vi "Acceleration Sensor-Dual.vi"() -> ()   [LabVIEW 2009]
uses:
  <vilib>/NXT/Block Support/NXT_InputPort.ctl
  <vilib>/NXT/Subs/LVHSConnector.ctl
  mindsensors.com LVEE Toolkit/Dual/Acceleration Sensor-DM.vi
panel:
  out "Status (boolean)":bool
  in  "stop":bool
  out "Z":i16(knob)=231 scale=-2000.0..2000.0
  out "Y":i16(knob) scale=-2000.0..2000.0
  out "X":i16(knob)=234 scale=-2000.0..2000.0
  out "X":i16(slide)=126 scale=-35.0..35.0
  out "Z":i16(slide)=129 caption="Y" scale=-35.0..35.0
  out "Y":i16(slide)=128 scale=-35.0..35.0
  out "Z":i16(slide)=125 caption="X" scale=-35.0..35.0
  out "Y 3":i16(slide)=128 caption="Y" scale=-35.0..35.0
  out "X":i16(slide)=126 scale=-35.0..35.0
  out "Z":dbl
  out "Y":dbl
  out "X":dbl
  out "Z":dbl=128.0
  out "Y  5":dbl=128.0
  out "X":dbl=128.0
  out "NXT dup":T1={"error"={"status"=FALSE, "code"=0, "source"=""}, "address"="", "NXT #"=-1, "Show Error"=TRUE} caption="NXT"
  in  "NXT":T1={"error"={"status"=FALSE, "code"=0, "source"=""}, "address"="", "NXT #"=-1, "Show Error"=TRUE}
  in  "Input Port":T2 items=["Port 1", "Port 2", "Port 3", "Port 4"]
  # "Tilt"
  # "Acceleration"
  # "mindsensors.com\nCopyright (c) 2009 by mindsensors.com\nEmail: info (<at>) mindsensors (<dot>) com\n\nThis program is free software. You can redistribute it and/or modify\nit under the terms of the GNU General Public License as published by\nthe Free Software Foundation; version 3 of the License.\nRead the license at: http://www.gnu.org/licenses/gpl.txt"
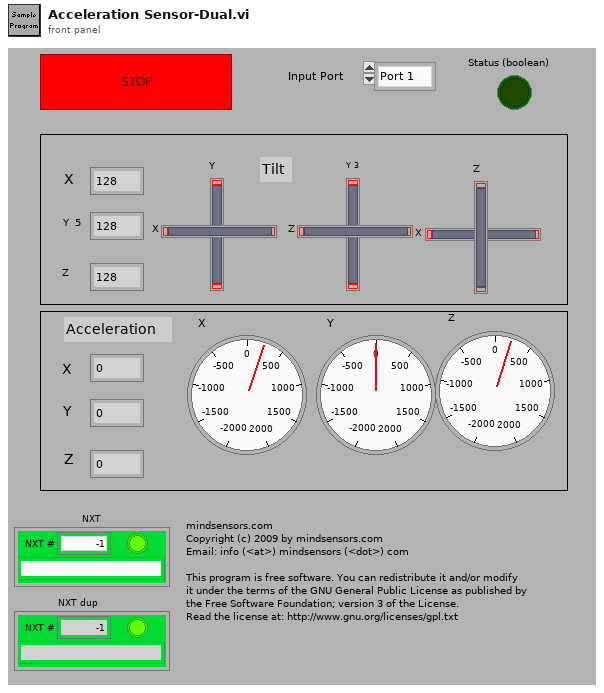
[diagram p1: front panel]
types:
  T1 = typedef "LVHSConnector.ctl" = cluster{"error":errorcluster, "address":string, "NXT #":i32, "Show Error":bool}
  T2 = typedef "NXT_InputPort.ctl" = u8
  T3 = cluster{"X Tilt":i16, "Y Tilt":i16, "Z Tilt":i16, "X Accel":i16, "Y Accel":i16, "Z Accel":i16, "Status (boolean)":bool}
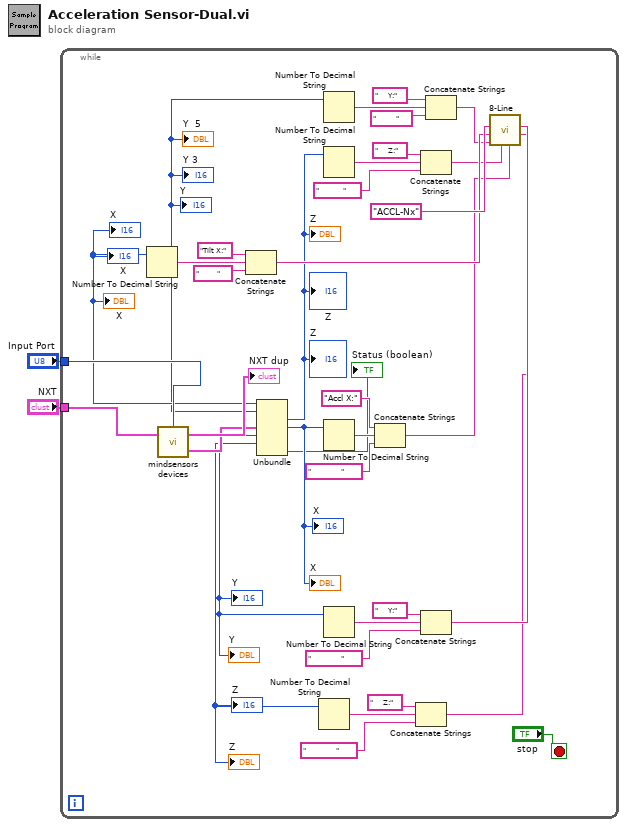
[diagram p0: block diagram]
diagram:
  n1 = while {
    tunnel: "Input Port" -> [w14]
    tunnel: "NXT" -> [w13]
    stop <- "stop" stop-if-true
    n2 = call-poly "mindsensors devices.vi"("NXT"=w13, "Input Port"=w14) -> ("Output of Acceleration Sensor"=w11:T3, "NXT dup"=→"NXT dup":T1)  [unwired: 1 in]
    n3 = Unbundle(w11) -> ("X Tilt"=w10:i16, "Y Tilt"=w9:i16, "Z Tilt"=w8:i16, "X Accel"=w7:i16, "Y Accel"=w6:i16, "Z Accel"=w5:i16, "Status (boolean)"=→"Status (boolean)":bool)
    "X" <- w10
    "Y  5" <- w9
    "Z" <- w8
    "X" <- w7
    "Y" <- w6
    "Z" <- w5
    "X" <- w10
    "Y 3" <- w9
    "Z" <- w8
    "Y" <- w9
    "Z" <- w8
    "X" <- w10
    "X" <- w7
    "Y" <- w6
    "Z" <- w5
    n4 = Number To Decimal String(number=w10) -> (decimal integer string=w37:string)  [unwired: 1 in]
    n5 = Concatenate Strings("Tilt X:" ("string"), w37, "         " ("string")) -> (w36:string)
    n6 = Number To Decimal String(number=w5) -> (decimal integer string=w30:string)  [unwired: 1 in]
    n7 = Number To Decimal String(number=w9) -> (decimal integer string=w28:string)  [unwired: 1 in]
    n8 = Number To Decimal String(number=w8) -> (decimal integer string=w26:string)  [unwired: 1 in]
    n9 = Number To Decimal String(number=w7) -> (decimal integer string=w34:string)  [unwired: 1 in]
    n10 = Number To Decimal String(number=w6) -> (decimal integer string=w32:string)  [unwired: 1 in]
    n11 = Concatenate Strings("Accl X:" ("string"), w34, "               " ("string")) -> (w25:string)
    n12 = Concatenate Strings("     Z:" ("string"), w30, "               " ("string")) -> (w23:string)
    n13 = Concatenate Strings("     Z:" ("string"), w26, "            " ("string")) -> (w21:string)
    n14 = Concatenate Strings("     Y:" ("string"), w32, "               " ("string")) -> (w24:string)
    n15 = Concatenate Strings("     Y:" ("string"), w28, "          " ("string")) -> (w22:string)
    n16 = call "8-Line.vi"("Line 7"=w23, "Line 6"=w24, "Line 5"=w25, "Line 4"=w21, "Line 3"=w22, "Line 2"=w36, "Line 1"="ACCL-Nx") -> ()  [unwired: 4 in, 1 out]
  }
